vi "Status Steuerung.vi"() -> ()   [LabVIEW 2020, in "Erweiterte Konfig.lvlib"]
uses:
  Erweiterte Konfig.lvlib
  Visualisierungs Elemente/Button.ctl
  cRIO/Verwaltung/Digital Eingaenge 0-15.ctl
  cRIO/Verwaltung/Digital Ausgaenge 0-31.ctl
  cRIO/Verwaltung/Analog Eingaenge.ctl
  cRIO/Allgemein/CPU Status.ctl
  cRIO/Allgemein/CPU Speicher Auslastung.ctl
  cRIO/Verwaltung/Digital Ausgaenge 32-63.ctl
  cRIO/Verwaltung/TC Eingaenge.ctl
  <vilib>/Utility/miscctls.llb/LVRowAndColumnTypeDef.ctl
  System Load/VI SysLoad.vi
  cRIO/PC/Kommunikation mit cRIO.lvlib
  Allgemein/allgemeine Sub-VIs.lvlib
  System Load/System Load.lvlib
  cRIO/Verwaltung/Verwaltung - cRIO.lvlib
  cRIO/Allgemein/Allgemein.lvlib
panel:
  in  "Hauptregisterkarte":T1(tab)
  out "Digital In 2":string[][](table) caption="Digital In"
  out "Digital In":string[][](table)
  out "Digital Out 2":string[][](table) caption="Digital Out 1"
  out "Digital Out 1":string[][](table)
  out "Analog In 2":string[][](table) caption="Analog In"
  out "Analog In":string[][](table)
  out "TC In 2":string[][](table)
  out "TC In 1":string[][](table)
  out "PID":string[][](table)=[["Heizung Filter:"], ["Heizung Pumpe:"], ["Heizung HL zu Filter:"], ["Heizung HL zu FT-IR:"], ["HL zu FID:"], ["Reserve"], ["Heizleitung SP1:"], ["Heizleitung SP2:"], ["Flussregelung"], ["Reserve:"], [""], [""]]
  in  "Systemauslastung":T2
  in  "Registerkarte":T3(tab)
  out "DI":T4
  out "DO":T5
  out "DO 32-63":T6
  out "Analog Input":T7
  out "TC Eingänge":T8
  out "CPU Auslastung":T9 caption="CPU usage"
  out "CPU Speicher":T10 caption="CPU memory"
  out "PID Stellwerte":i16[](array[numeric]) caption="Controller Output"
  in  "ABBRECHEN":T2
  # "Status PLC"
  # "Heating filter:"
  # "Heating Pump:"
  # "Heating HL to filter:"
  # "Heating HL to FT-IR:"
  # "HL zu FID:"
  # "Reserve"
  # "Heizleitung SP1:"
  # "Heizleitung SP2:"
  # "Flussregelung"
  # "Option:"
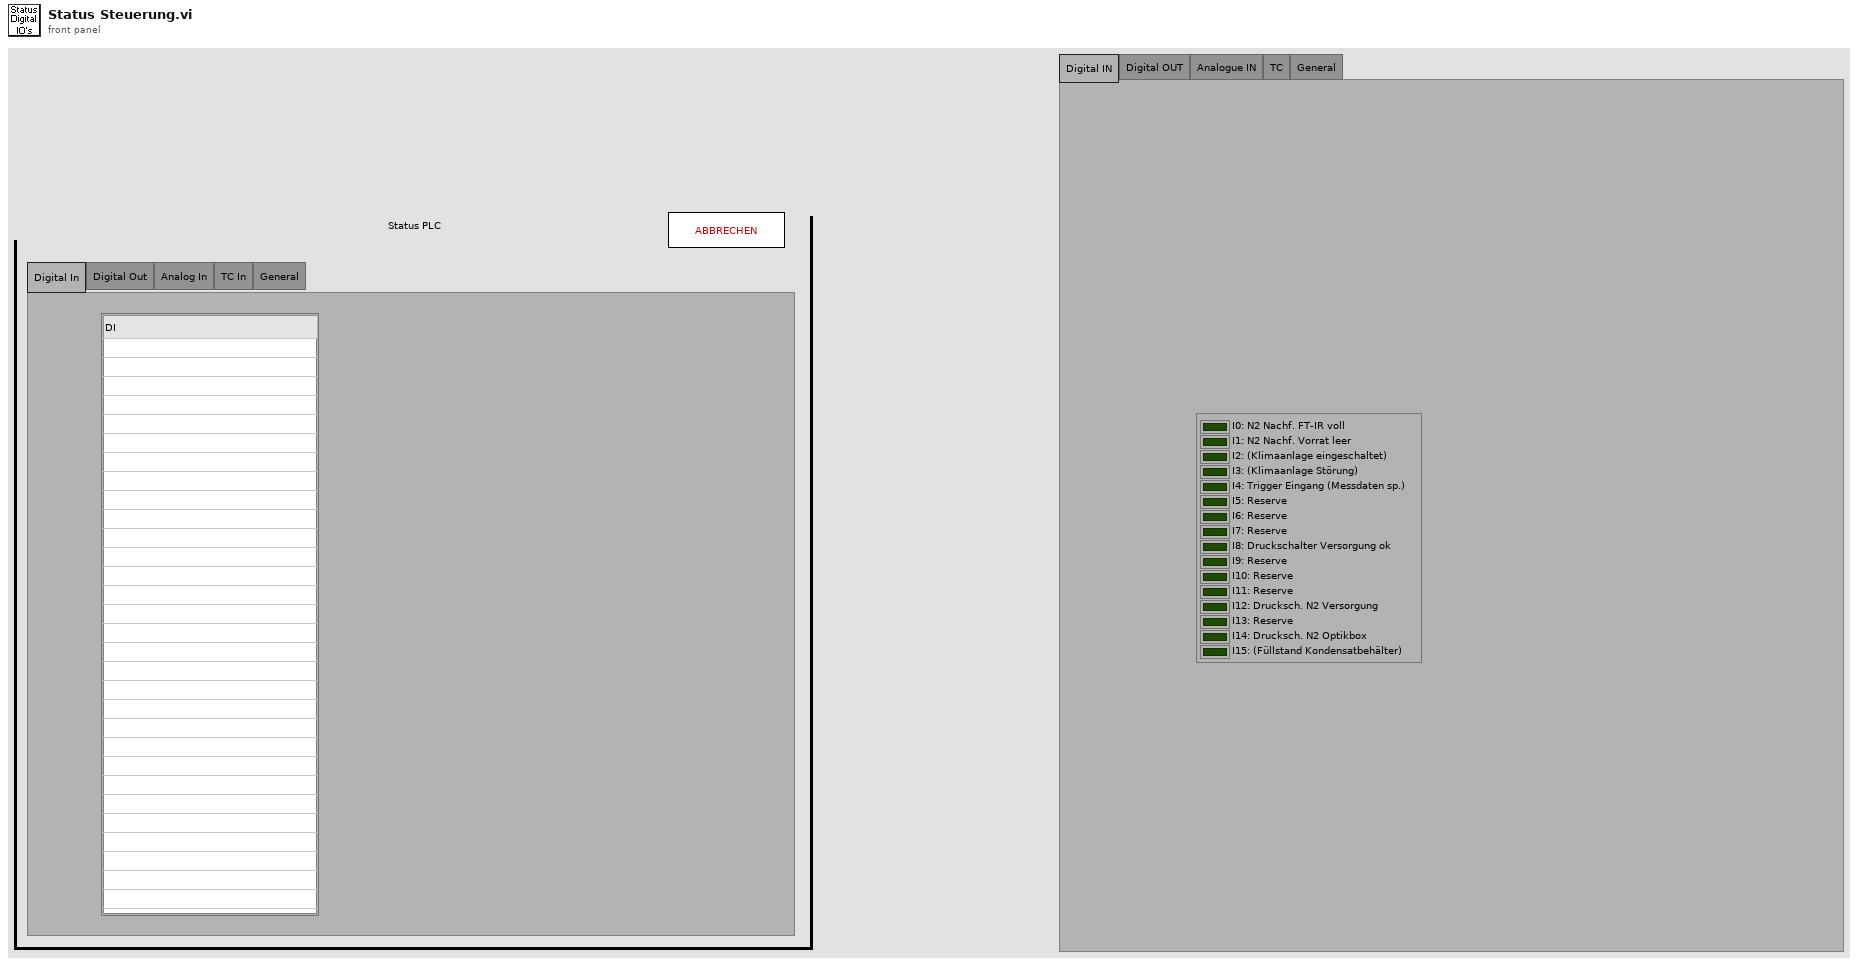
[diagram p1: front panel]
types:
  T1 = enum32{"Digital In", "Digital Out", "Analog In", "TC In", "General", "HovaCal Einstellungen"}
  T2 = typedef "Button.ctl" = bool
  T3 = enum32{"Digital IN", "Digital OUT", "Analogue IN", "TC", "General"}
  T4 = typedef "Verwaltung - cRIO.lvlib/Digital Eingaenge 0-15.ctl" = cluster{"I0: N2 Nachf. FT-IR voll":bool, "I1: N2 Nachf. Vorrat leer":bool, "I2: (Klimaanlage eingeschaltet)":bool, "I3: (Klimaanlage Störung)":bool, "I4: Trigger Eingang (Messdaten sp.)":bool, "I5: Reserve":bool, "I6: Reserve":bool, "I7: Reserve":bool, "I8: Druckschalter Versorgung ok":bool, "I9: Reserve":bool, "I10: Reserve":bool, "I11: Reserve":bool, "I12: Drucksch. N2 Versorgung":bool, "I13: Reserve":bool, "I14: Drucksch. N2 Optikbox":bool, "I15: (Füllstand Kondensatbehälter)":bool}
  T5 = typedef "Verwaltung - cRIO.lvlib/Digital Ausgaenge 0-31.ctl" = cluster{"O0: Druckluft Versorgung":bool, "O1: CG 1 (FB Eingang 1)":bool, "O2: CG 2 (Kühlung FT-IR EIN)":bool, "O3: CG 3 (FB Bypass)":bool, "O4: CG 4 (FB CalGas)":bool, "O5: CG 5 (FB spülen/UL)":bool, "O6: CG 6 (FB zum FT-IR)":bool, "O7: CG 7 (FB zum FID)":bool, "O8: CG 8 (FB Reserve)":bool, "O9: (FB Reserve)":bool, "O10: (FB Umgebungsluft FID)":bool, "O11: (FB zum Gaskühler)":bool, "O12: FB Stickstoff zu FT-IR":bool, "O13: Optikbox FT-IR spülen":bool, "O14: (Purifier deaktivieren)":bool, "O15: (Umschaltung Purifier/Stickstoff)":bool, "O16: N2 Einblasung":bool, "O17: LSP LN2 Nachfüllung":bool, "O18: (Reserve)":bool, "O19: (Pumpe Eingang1)":bool, "O20: (Pumpe Eingang2)":bool, "O21: (Pumpe Spülen1)":bool, "O22: (Pumpe Spülen2)":bool, "O23: (Reserve)":bool, "O24: CalGas 1":bool, "O25: CalGas 2":bool, "O26: CG 3-8 (CalGas 3)":bool, "O27: Stickstoff aufschalten":bool, "O28: CG zu PNS":bool, "O29: FTIR Standby Spülung":bool, "O30: CG zu Entnahme(T90)":bool, "O31: (Purifier regenerieren)":bool}
  T6 = typedef "Verwaltung - cRIO.lvlib/Digital Ausgaenge 32-63.ctl" = cluster{"O32: Messgaspumpe EIN":bool, "O33: (Umgebungsluftpumpe)":bool, "O34: (Kondensatpumpe GK)":bool, "O35: Klima/Lüfter EIN":bool, "O36: Versorgung Heizungen":bool, "O37: Versorgung Heizungen":bool, "O38: (Gaskühler EIN (Freigabe))":bool, "O39: Störung FAS LP":bool, "O40: (Heizung Filterblock)":bool, "O41: Heizung HL zu FT-IR":bool, "O42: Heizung HL Extern SP1":bool, "O43: Heizung HL Extern SP2":bool, "O44: Heizung Reserve":bool, "O45: Heizung Reserve":bool, "O46: Statusbeleuchtung grün":bool, "O47: Statusbeleuchtung rot":bool}
  T7 = typedef "Verwaltung - cRIO.lvlib/Analog Eingaenge.ctl" = cluster{"AI0: Durchfluss FT-IR":sgl, "AI1: Druck Ausgang":sgl, "AI2: Umgebungsdruck":sgl, "AI3: Druck FT-IR":sgl, "AI4: Druck CalGas":sgl, "AI5: Reserve":sgl, "AI6: Reserve":sgl, "AI7: Reserve":sgl, "Rohwert Durchfluss FT-IR":sgl, "Rohwert Druck Ausgang":sgl, "Rohwert Umgebungsdruck":sgl, "Rohwert Druck FT-IR":sgl, "Rohwert Druck CalGas":sgl, "Rohwert AI5":sgl, "Rohwert AI6":sgl, "Rohwert AI7":sgl, "Rohwert Diffdruck mbar FTIR":sgl}
  T8 = typedef "Verwaltung - cRIO.lvlib/TC Eingaenge.ctl" = cluster{"TC0: Reserve":sgl, "TC1: HL zu FT-IR":sgl, "TC2: HL Extern SP1":sgl, "TC3: HL Extern SP2":sgl, "TC4: Reserve":sgl, "TC5: Reserve":sgl, "TC6: Reserve":sgl, "TC7: Reserve":sgl, "TC8: FT-IR":sgl, "TC9: Reserve":sgl, "TC10: Schaltschrank":sgl, "TC11: Umgebung":sgl}
  T9 = typedef "Allgemein.lvlib/CPU Status.ctl" = cluster{"Total (%)":sgl, "Time Critical (%)":sgl, "Timed Structures (%)":sgl, "High (%)":sgl, "Above Normal (%)":sgl, "Normal (%)":sgl, "Background (%)":sgl, "Idle (%)":sgl, "ISR (%)":sgl}
  T10 = typedef "Allgemein.lvlib/CPU Speicher Auslastung.ctl" = cluster{"total (bytes)":u32, "available (bytes)":u32, "largest contiguous (bytes)":u32}
  T11 = typedef "LVRowAndColumnTypeDef.ctl" = cluster{"Row":i32, "Column":i32}
  T12 = cluster{"Numeric":sgl, "Numeric":sgl, "Numeric":sgl, "Numeric":sgl, "Numeric":sgl, "Numeric":sgl, "Numeric":sgl, "Numeric":sgl, "Numeric":sgl}
  T13 = cluster{"Numeric":sgl, "Numeric":sgl, "Numeric":sgl}
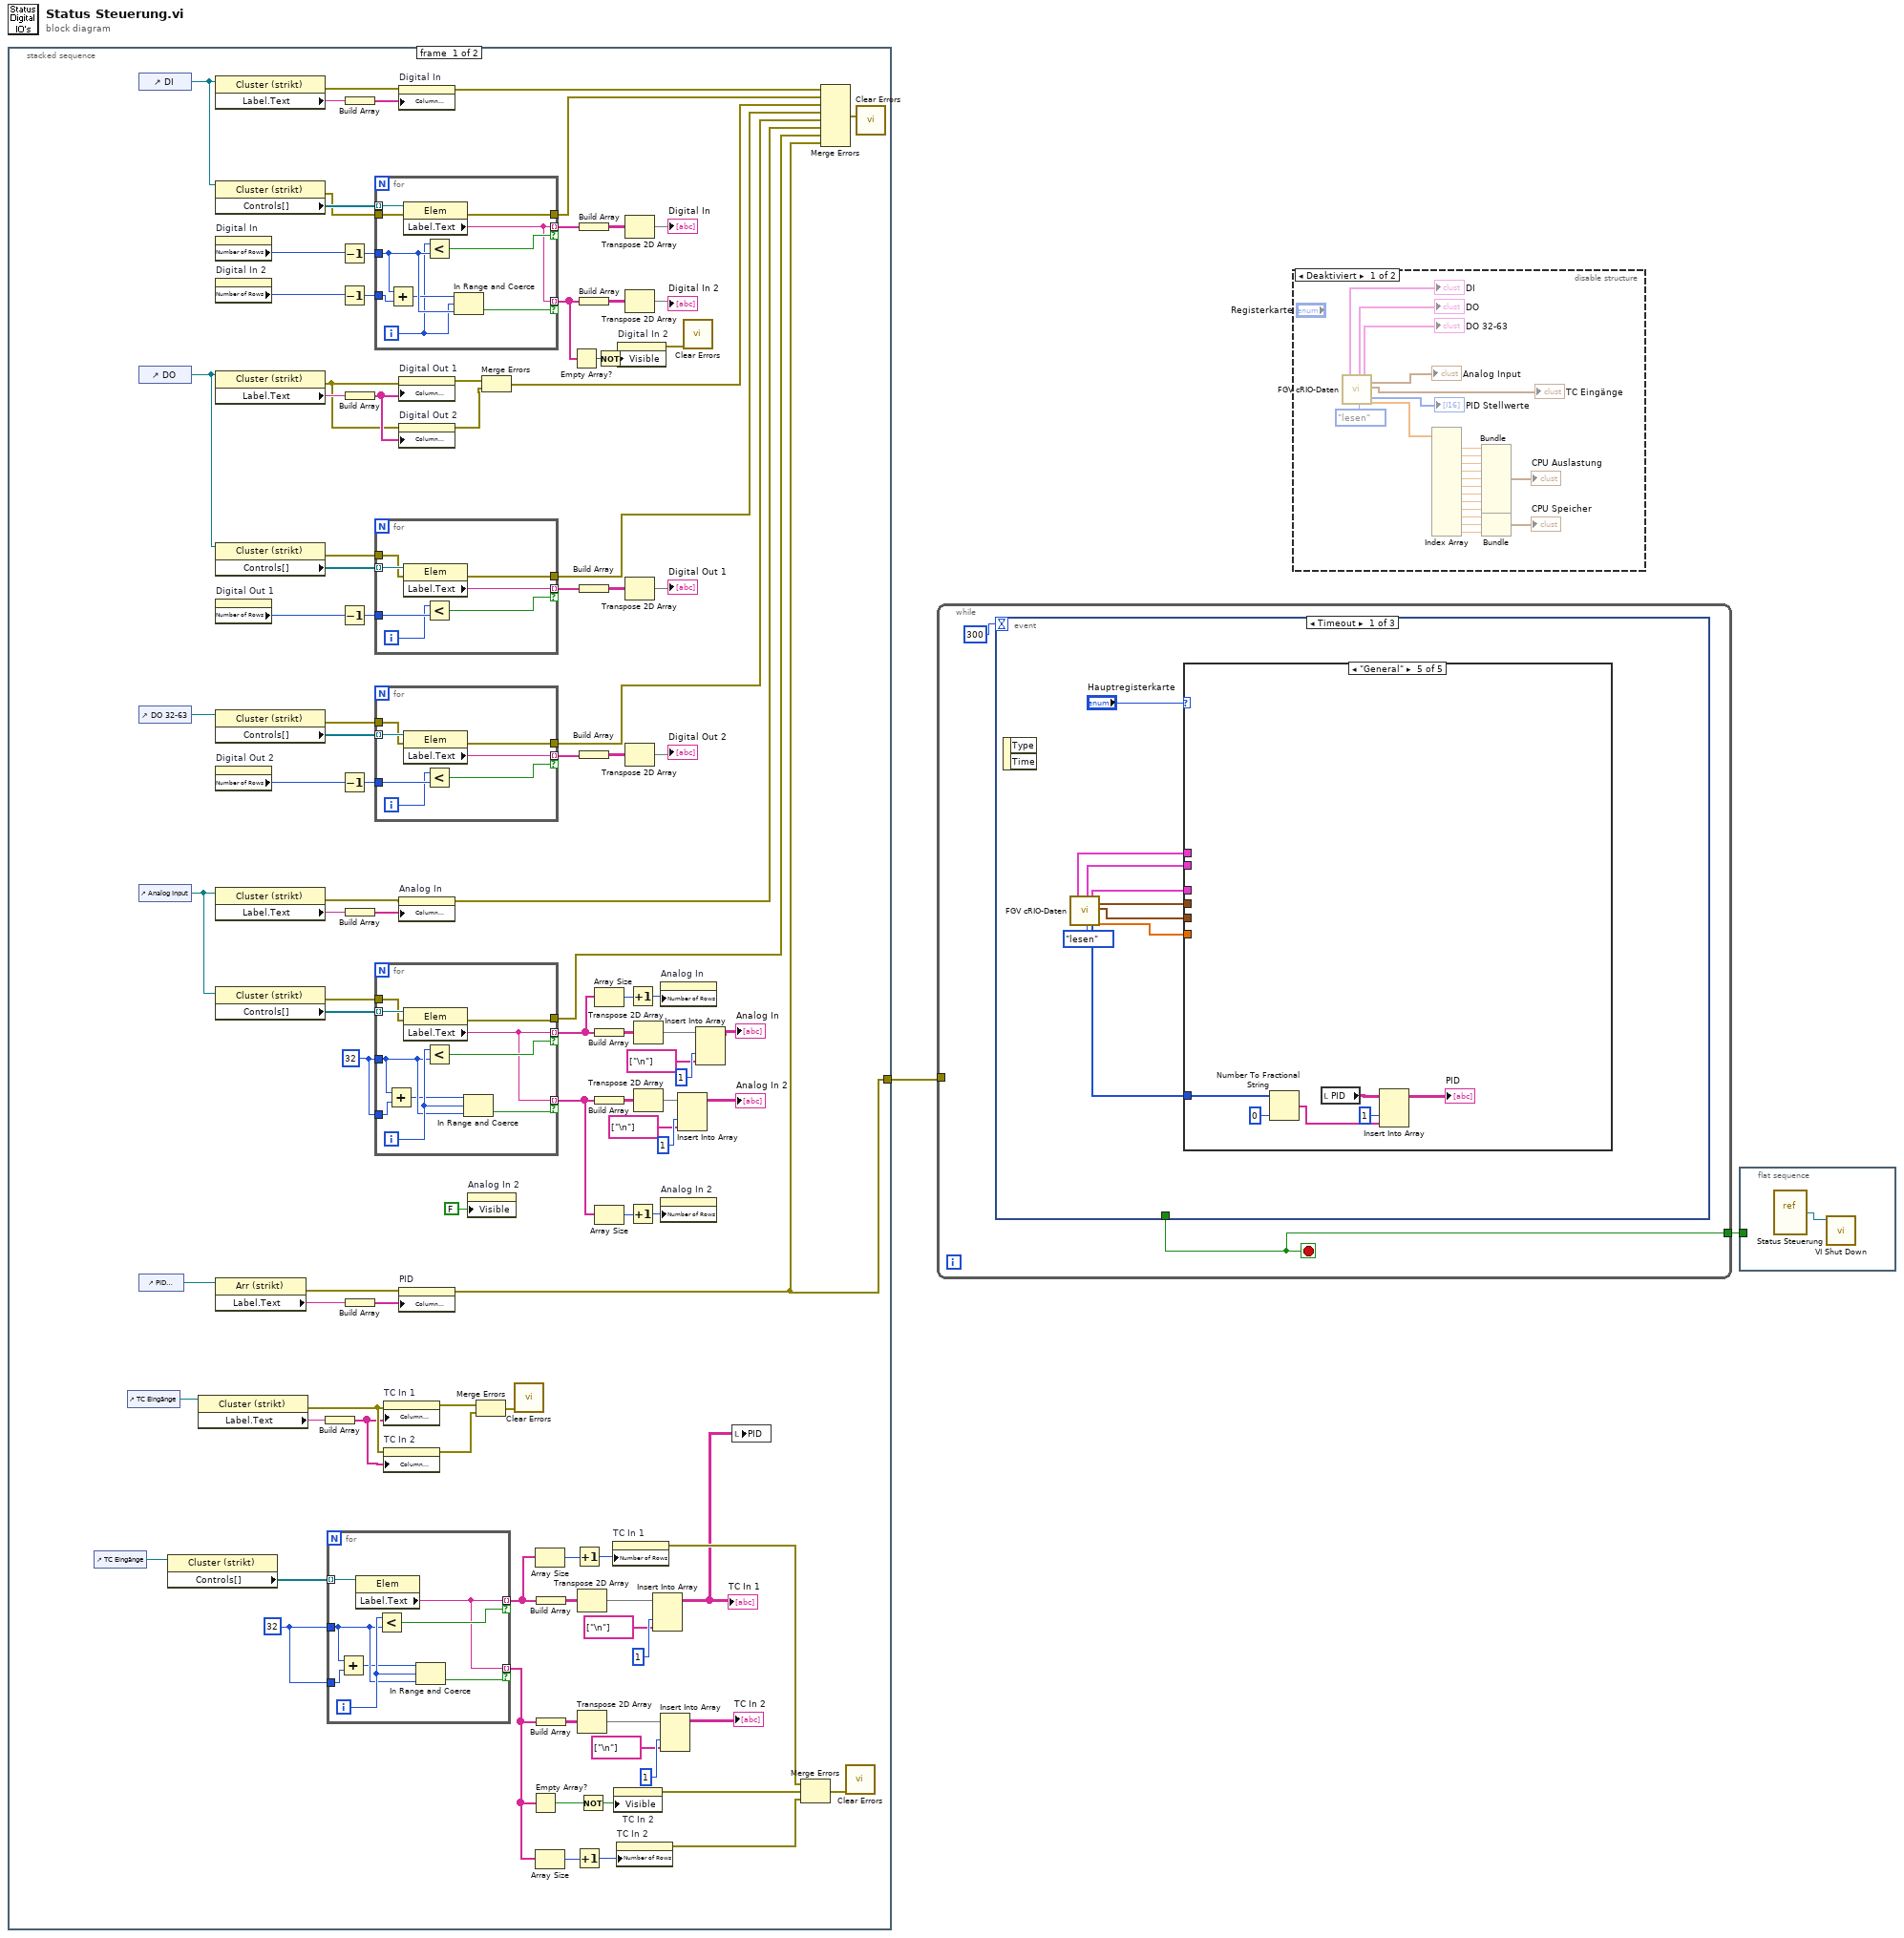
[diagram p0: block diagram]
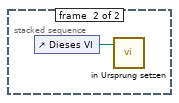
[diagram p3: hidden frame]
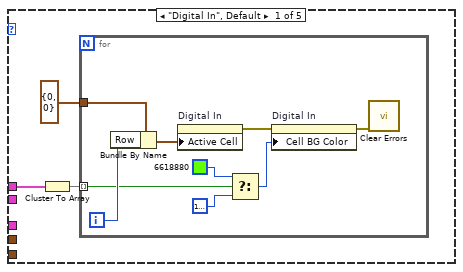
[diagram p4: hidden frame]
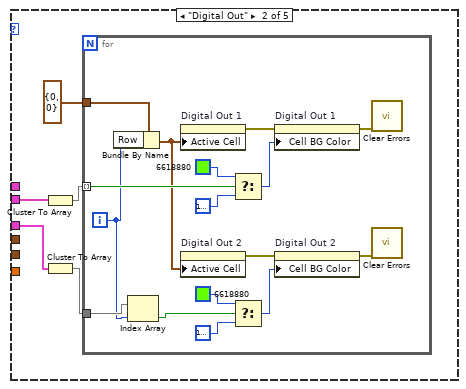
[diagram p5: hidden frame]
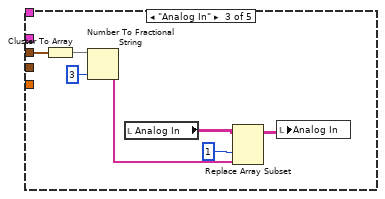
[diagram p6: hidden frame]
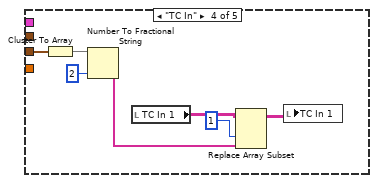
[diagram p7: hidden frame]
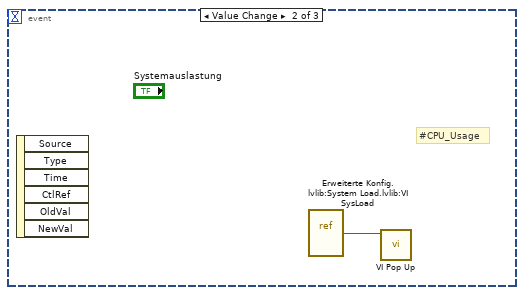
[diagram p8: hidden frame]
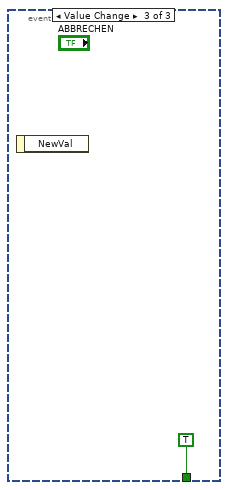
[diagram p9: hidden frame]
diagram:
  n1 = stacked-sequence {
    tunnel: [w5 _] -> w1
    frame #0 {
      w32 = u32 32 ("Zeilenanzahl")
      w43 = u32 32
      n2 = control-ref of="TC Eingänge"() -> (w74:refnum<vi>)
      n3 = control-ref of="TC Eingänge"() -> (w79:refnum<vi>)
      n4 = control-ref of="DI"() -> (w65:refnum<vi>)
      n5 = control-ref of="DO"() -> (w64:refnum<vi>)
      n6 = control-ref of="DO 32-63"() -> (w96:refnum<vi>)
      n7 = control-ref of="Analog Input"() -> (w63:refnum<vi>)
      n8 = control-ref of="PID Stellwerte"() -> (w66:refnum<vi>)
      n9 = property class="Cluster (strikt)"(reference=w74) -> ("Controls[]"=w76:refnum<vi>[])  [unwired: 1 in, 2 out]
      n10 = property class="Cluster (strikt)"(reference=w79) -> (error out=w81:errorcluster, "Label.Text"=w78:string)  [unwired: 1 in, 1 out]
      n11 = property class="Cluster (strikt)"(reference=w65) -> (error out=w89:errorcluster, "Label.Text"=w108:string)  [unwired: 1 in, 1 out]
      n12 = property class="Cluster (strikt)"(reference=w65) -> (error out=w62:errorcluster, "Controls[]"=w111:refnum<vi>[])  [unwired: 1 in, 1 out]
      n13 = property on="Digital In" class="Tbl (strikt)"() -> ("Number of Rows"=w90:u32)  [unwired: 2 in, 2 out]
      n14 = property on="Digital In 2" class="Tbl (strikt)"() -> ("Number of Rows"=w71:u32)  [unwired: 2 in, 2 out]
      n15 = property class="Cluster (strikt)"(reference=w64) -> (error out=w98:errorcluster, "Label.Text"=w106:string)  [unwired: 1 in, 1 out]
      n16 = property class="Cluster (strikt)"(reference=w64) -> (error out=w61:errorcluster, "Controls[]"=w101:refnum<vi>[])  [unwired: 1 in, 1 out]
      n17 = property on="Digital Out 1" class="Tbl (strikt)"() -> ("Number of Rows"=w104:u32)  [unwired: 2 in, 2 out]
      n18 = property class="Cluster (strikt)"(reference=w96) -> (error out=w60:errorcluster, "Controls[]"=w95:refnum<vi>[])  [unwired: 1 in, 1 out]
      n19 = property on="Digital Out 2" class="Tbl (strikt)"() -> ("Number of Rows"=w94:u32)  [unwired: 2 in, 2 out]
      n20 = property class="Cluster (strikt)"(reference=w63) -> (error out=w86:errorcluster, "Label.Text"=w85:string)  [unwired: 1 in, 1 out]
      n21 = property class="Cluster (strikt)"(reference=w63) -> (error out=w59:errorcluster, "Controls[]"=w83:refnum<vi>[])  [unwired: 1 in, 1 out]
      n22 = property class="Arr (strikt)"(reference=w66) -> (error out=w68:errorcluster, "Label.Text"=w69:string)  [unwired: 1 in, 1 out]
      n23 = Build Array(w78) -> (w80:string[])
      n24 = for {
        tunnel: w76 -> [w119] mode=indexing
        tunnel: [w113] -> w42 mode=indexing if=w118
        tunnel: w43 -> [w115]
        tunnel: w43 -> [w116]
        tunnel: [w113] -> w33 mode=indexing if=w112
        i -> [w117]
        n25 = Add(x=w115, y=w116) -> (x+y=w114:u32)
        n26 = property class="Elem"(reference=w119) -> ("Label.Text"=w113:string)  [unwired: 1 in, 2 out]
        n27 = Less?(x=w117, y=w115) -> (x < y?=w118:bool)
        n28 = In Range and Coerce(upper limit=w114, x=w117, lower limit=w115) -> (In Range?=w112:bool)  [unwired: 1 out]
      }
      n29 = Decrement(x=w90) -> (x-1=w107:u32)
      n30 = Decrement(x=w71) -> (x-1=w70:u32)
      n31 = Decrement(x=w104) -> (x-1=w105:u32)
      n32 = Decrement(x=w94) -> (x-1=w93:u32)
      n33 = Build Array(w108) -> (w88:string[])
      n34 = Build Array(w106) -> (w99:string[])
      n35 = Build Array(w85) -> (w87:string[])
      n36 = Build Array(w69) -> (w67:string[])
      n37 = for {
        tunnel: w111 -> [w153] mode=indexing
        tunnel: [w151] -> w110 mode=indexing if=w152
        tunnel: w107 -> [w148]
        tunnel: [w151] -> w49 mode=indexing if=w150
        tunnel: w70 -> [w149]
        tunnel: w62 -> [w145]
        tunnel: [w144] -> w57
        i -> [w146]
        n38 = Add(x=w148, y=w149) -> (x+y=w147:u32)
        n39 = property class="Elem"(reference=w153, error in=w145) -> (error out=w144:errorcluster, "Label.Text"=w151:string)  [unwired: 1 out]
        n40 = Less?(x=w146, y=w148) -> (x < y?=w152:bool)
        n41 = In Range and Coerce(upper limit=w147, x=w146, lower limit=w148) -> (In Range?=w150:bool)  [unwired: 1 out]
      }
      n42 = for {
        tunnel: w101 -> [w143] mode=indexing
        tunnel: [w142] -> w102 mode=indexing if=w141
        tunnel: w105 -> [w140]
        tunnel: w61 -> [w138]
        tunnel: [w137] -> w53
        i -> [w139]
        n43 = property class="Elem"(reference=w143, error in=w138) -> (error out=w137:errorcluster, "Label.Text"=w142:string)  [unwired: 1 out]
        n44 = Less?(x=w139, y=w140) -> (x < y?=w141:bool)
      }
      n45 = for {
        tunnel: w95 -> [w136] mode=indexing
        tunnel: [w135] -> w92 mode=indexing if=w134
        tunnel: w93 -> [w133]
        tunnel: w60 -> [w131]
        tunnel: [w130] -> w52
        i -> [w132]
        n46 = property class="Elem"(reference=w136, error in=w131) -> (error out=w130:errorcluster, "Label.Text"=w135:string)  [unwired: 1 out]
        n47 = Less?(x=w132, y=w133) -> (x < y?=w134:bool)
      }
      n48 = for {
        tunnel: w83 -> [w129] mode=indexing
        tunnel: [w123] -> w30 mode=indexing if=w128
        tunnel: w32 -> [w125]
        tunnel: w32 -> [w126]
        tunnel: [w123] -> w28 mode=indexing if=w122
        tunnel: w59 -> [w121]
        tunnel: [w120] -> w50
        i -> [w127]
        n49 = Add(x=w125, y=w126) -> (x+y=w124:u32)
        n50 = property class="Elem"(reference=w129, error in=w121) -> (error out=w120:errorcluster, "Label.Text"=w123:string)  [unwired: 1 out]
        n51 = Less?(x=w127, y=w125) -> (x < y?=w128:bool)
        n52 = In Range and Coerce(upper limit=w124, x=w127, lower limit=w125) -> (In Range?=w122:bool)  [unwired: 1 out]
      }
      n53 = property on="TC In 1" class="Tbl (strikt)"(error in=w81, "Column Headers[]"=w80) -> (error out=w24:errorcluster)  [unwired: 1 in, 1 out]
      n54 = property on="TC In 2" class="Tbl (strikt)"(error in=w81, "Column Headers[]"=w80) -> (error out=w23:errorcluster)  [unwired: 1 in, 1 out]
      n55 = property on="Digital In" class="Tbl (strikt)"(error in=w89, "Column Headers[]"=w88) -> (error out=w58:errorcluster)  [unwired: 1 in, 1 out]
      n56 = property on="Digital Out 1" class="Tbl (strikt)"(error in=w98, "Column Headers[]"=w99) -> (error out=w56:errorcluster)  [unwired: 1 in, 1 out]
      n57 = property on="Digital Out 2" class="Tbl (strikt)"(error in=w98, "Column Headers[]"=w99) -> (error out=w55:errorcluster)  [unwired: 1 in, 1 out]
      n58 = property on="Analog In" class="Tbl (strikt)"(error in=w86, "Column Headers[]"=w87) -> (error out=w51:errorcluster)  [unwired: 1 in, 1 out]
      n59 = property on="PID" class="Tbl (strikt)"(error in=w68, "Column Headers[]"=w67) -> (error out=w5:errorcluster)  [unwired: 1 in, 1 out]
      n60 = property on="Analog In 2" class="Tbl (strikt)"("Visible"=FALSE ("Sichtbar")) -> ()  [unwired: 2 in, 2 out]
      n61 = Merge Errors(w24, w23) -> (w22:errorcluster)
      n62 = Merge Errors(w56, w55) -> (w54:errorcluster)
      n63 = call <vilib>:"Clear Errors.vi"("error in (no error)"=w22) -> ()  [unwired: 5 in, 2 out]
      n64 = Empty Array?(array=w33) -> (empty?=w45:bool)
      n65 = Array Size(array=w42) -> (size(s)=w41:i32)
      n66 = Array Size(array=w33) -> (size(s)=w35:i32)
      n67 = Build Array(w42) -> (w75:string[][])
      n68 = Build Array(w33) -> (w77:string[][])
      n69 = Empty Array?(array=w49) -> (empty?=w48:bool)
      n70 = Increment(x=w41) -> (x+1=w40:i32)
      n71 = Increment(x=w35) -> (x+1=w34:i32)
      n72 = Transpose 2D Array(2D array=w75) -> (transposed array=w10:string[][])
      n73 = Transpose 2D Array(2D array=w77) -> (transposed array=w7:string[][])
      n74 = Not(x=w45) -> (.not. x?=w44:bool)
      n75 = Build Array(w110) -> (w109:string[][])
      n76 = Build Array(w49) -> (w73:string[][])
      n77 = Build Array(w102) -> (w103:string[][])
      n78 = Build Array(w92) -> (w97:string[][])
      n79 = Array Size(array=w30) -> (size(s)=w31:i32)
      n80 = Build Array(w30) -> (w84:string[][])
      n81 = Build Array(w28) -> (w82:string[][])
      n82 = Array Size(array=w28) -> (size(s)=w29:i32)
      n83 = Not(x=w48) -> (.not. x?=w46:bool)
      n84 = property on="TC In 1" class="Tbl (strikt)"("Number of Rows"=w40) -> (error out=w38:errorcluster)  [unwired: 2 in, 1 out]
      n85 = property on="TC In 2" class="Tbl (strikt)"("Visible"=w44) -> (error out=w37:errorcluster)  [unwired: 2 in, 1 out]
      n86 = property on="TC In 2" class="Tbl (strikt)"("Number of Rows"=w34) -> (error out=w36:errorcluster)  [unwired: 2 in, 1 out]
      n87 = property on="Digital In 2" class="Tbl (strikt)"("Visible"=w46) -> (error out=w47:errorcluster)  [unwired: 2 in, 1 out]
      n88 = Transpose 2D Array(2D array=w109) -> (transposed array=→"Digital In":string[][])
      n89 = Transpose 2D Array(2D array=w73) -> (transposed array=→"Digital In 2":string[][])
      n90 = Transpose 2D Array(2D array=w103) -> (transposed array=→"Digital Out 1":string[][])
      n91 = Transpose 2D Array(2D array=w97) -> (transposed array=→"Digital Out 2":string[][])
      n92 = Increment(x=w31) -> (x+1=w26:i32)
      n93 = Increment(x=w29) -> (x+1=w27:i32)
      n94 = Transpose 2D Array(2D array=w84) -> (transposed array=w17:string[][])
      n95 = Transpose 2D Array(2D array=w82) -> (transposed array=w14:string[][])
      n96 = Insert Into Array(array=w10, index (col)=1 ("Deaktivierter Index (Spalte)"), new element=string[] ["\n"] ("Neues Element/Teil-Array")) -> (w3:string[][])  [unwired: 1 in]
      "TC In 1" <- w3
      n97 = property on="Analog In" class="Tbl (strikt)"("Number of Rows"=w26) -> ()  [unwired: 2 in, 2 out]
      n98 = property on="Analog In 2" class="Tbl (strikt)"("Number of Rows"=w27) -> ()  [unwired: 2 in, 2 out]
      n99 = Insert Into Array(array=w7, index (col)=1 ("Deaktivierter Index (Spalte)"), new element=string[] ["\n"] ("Neues Element/Teil-Array")) -> (→"TC In 2":string[][])  [unwired: 1 in]
      n100 = Insert Into Array(array=w14, index (col)=1 ("Deaktivierter Index (Spalte)"), new element=string[] ["\n"] ("Neues Element/Teil-Array")) -> (→"Analog In 2":string[][])  [unwired: 1 in]
      n101 = call <vilib>:"Clear Errors.vi"("error in (no error)"=w47) -> ()  [unwired: 5 in, 2 out]
      n102 = Insert Into Array(array=w17, index (col)=1 ("Deaktivierter Index (Spalte)"), new element=string[] ["\n"] ("Neues Element/Teil-Array")) -> (→"Analog In":string[][])  [unwired: 1 in]
      n103 = local write "PID"(w3) -> ()
      n104 = Merge Errors(w38, w37, w36) -> (w39:errorcluster)
      n105 = Merge Errors(w58, w57, w54, w53, w52, w51, w50, w5) -> (w21:errorcluster)
      n106 = call <vilib>:"Clear Errors.vi"("error in (no error)"=w39) -> ()  [unwired: 5 in, 2 out]
      n107 = call <vilib>:"Clear Errors.vi"("error in (no error)"=w21) -> ()  [unwired: 5 in, 2 out]
    }
    frame #1 {
      n108 = control-ref of="Dieses VI"() -> (w154:refnum<vi>)
      n109 = call "in Ursprung setzen.vi"("VI Referenz"=w154) -> ()  [unwired: 10 in, 1 out]
    }
  }
  n110 = while {
    tunnel: [w155] -> w2
    tunnel: w1 -> [_]
    stop <- w155 stop-if-true
    n111 = event shown="[0] Timeout" {
      selector: _ -> [_ _ _]
      dyn-events: _ -> [_ _ _]
      timeout: 300 -> [_ _ _]
      tunnel: [_ _ TRUE ("ABBRECHEN")] -> w155
      event Timeout {
        n112 = event-data() -> ()  [unwired: 1 in, 2 out]
        n113 = call "FGV cRIO-Daten.vi"("Aktion"=enum16{"lesen", "schreiben"}."lesen") -> ("DI"=w161:T4, "DO 0-31"=w162:T5, "DO 32-63"=w163:T6, "PID Stellwerte"=w157:i16[], "Analog Input"=w164:T7, "TC Eingänge"=w165:T8, "CPU Status"=w158:sgl[])  [unwired: 9 in, 3 out]
        n114 = case shown="\"General\"" "Hauptregisterkarte" {
          tunnel: w161 -> [w168 _ _ _ _]
          tunnel: w162 -> [_ w180 _ _ _]
          tunnel: w163 -> [_ w179 _ _ _]
          tunnel: w164 -> [_ _ w205 _ _]
          tunnel: w165 -> [_ _ _ w211 _]
          tunnel: w158 -> [_ _ _ _ _]
          tunnel: w157 -> [_ _ _ _ w218]
          frame "Digital In", Default {
            n115 = Cluster To Array(cluster=w168) -> (array=w167:bool[])
            n116 = for {
              tunnel: w167 -> [w173] mode=indexing
              tunnel: T11 {"Row"=0, "Column"=0} ("Aktive Zelle:Aktive Zelle") -> [w177]
              i -> [w176]
              n117 = Bundle By Name(cluster=w177, "Row"=w176) -> (w175:T11)
              n118 = property on="Digital In" class="Tbl (strikt)"("Active Cell"=w175) -> (error out=w174:errorcluster)  [unwired: 2 in, 1 out]
              n119 = Select(t=u32 6618880, s=w173, f=u32 16777225) -> (s? t:f=w172:u32)
              n120 = property on="Digital In" class="Tbl (strikt)"(error in=w174, "Cell BG Color"=w172) -> (error out=w171:errorcluster)  [unwired: 1 in, 1 out]
              n121 = call <vilib>:"Clear Errors.vi"("error in (no error)"=w171) -> ()  [unwired: 5 in, 2 out]
            }
          }
          frame "Digital Out" {
            n122 = Cluster To Array(cluster=w180) -> (array=w181:bool[])
            n123 = Cluster To Array(cluster=w179) -> (array=w178:bool[])
            n124 = for {
              tunnel: w181 -> [w192] mode=indexing
              tunnel: T11 {"Row"=0, "Column"=0} ("Aktive Zelle:Aktive Zelle") -> [w198]
              tunnel: w178 -> [w185]
              i -> [w183]
              n125 = Bundle By Name(cluster=w198, "Row"=w183) -> (w186:T11)
              n126 = Index Array(array=w185, index=w183) -> (element=w184:bool)
              n127 = property on="Digital Out 1" class="Tbl (strikt)"("Active Cell"=w186) -> (error out=w197:errorcluster)  [unwired: 2 in, 1 out]
              n128 = property on="Digital Out 2" class="Tbl (strikt)"("Active Cell"=w186) -> (error out=w187:errorcluster)  [unwired: 2 in, 1 out]
              n129 = Select(t=u32 6618880, s=w192, f=u32 16777225) -> (s? t:f=w196:u32)
              n130 = Select(t=u32 6618880, s=w184, f=u32 16777225) -> (s? t:f=w188:u32)
              n131 = property on="Digital Out 1" class="Tbl (strikt)"(error in=w197, "Cell BG Color"=w196) -> (error out=w195:errorcluster)  [unwired: 1 in, 1 out]
              n132 = property on="Digital Out 2" class="Tbl (strikt)"(error in=w187, "Cell BG Color"=w188) -> (error out=w189:errorcluster)  [unwired: 1 in, 1 out]
              n133 = call <vilib>:"Clear Errors.vi"("error in (no error)"=w195) -> ()  [unwired: 5 in, 2 out]
              n134 = call <vilib>:"Clear Errors.vi"("error in (no error)"=w189) -> ()  [unwired: 5 in, 2 out]
            }
          }
          frame "Analog In" {
            n135 = Cluster To Array(cluster=w205) -> (array=w204:sgl[])
            n136 = Number To Fractional String(number=w204, precision (6)=i16 3 ("Genauigkeit (6)")) -> (F-format string=w199:string[])  [unwired: 2 in]
            n137 = local read "Analog In"() -> (w200:string[][])
            n138 = Replace Array Subset(array=w200, new element=w199, index (col)=1 ("Deaktivierter Index (Spalte)")) -> (w201:string[][])  [unwired: 1 in]
            n139 = local write "Analog In"(w201) -> ()
          }
          frame "TC In" {
            n140 = Cluster To Array(cluster=w211) -> (array=w212:sgl[])
            n141 = Number To Fractional String(number=w212, precision (6)=i16 2 ("Genauigkeit (6)")) -> (F-format string=w206:string[])  [unwired: 2 in]
            n142 = local read "TC In 1"() -> (w208:string[][])
            n143 = Replace Array Subset(array=w208, new element=w206, index (col)=1 ("Deaktivierter Index (Spalte)")) -> (w207:string[][])  [unwired: 1 in]
            n144 = local write "TC In 1"(w207) -> ()
          }
          frame "General" {
            n145 = Number To Fractional String(number=w218, precision (6)=i16 0 ("Genauigkeit (6)")) -> (F-format string=w214:string[])  [unwired: 2 in]
            n146 = local read "PID"() -> (w216:string[][])
            n147 = Insert Into Array(array=w216, index (col)=1 ("Deaktivierter Index (Spalte)"), new element=w214) -> (→"PID":string[][])  [unwired: 1 in]
          }
        }
      }
      event Value Change {
        # "#CPU_Usage"
        n148 = event-data() -> ()  [unwired: 1 in, 6 out]
        n149 = vi-ref "Erweiterte Konfig.lvlib:System Load.lvlib:VI SysLoad.vi"() -> (w219:refnum<vi>)
        n150 = call "VI Pop Up.vi"("VI Referenz"=w219) -> ()  [unwired: 10 in, 1 out]
      }
      event Value Change {
        n151 = event-data() -> ()  [unwired: 1 in, 1 out]
      }
    }
  }
  n152 = disable-structure shown="Deaktiviert" {
    frame Disabled {
      n153 = call "FGV cRIO-Daten.vi"("Aktion"=enum16{"lesen", "schreiben"}."lesen") -> ("DI"=→"DI":T4, "DO 0-31"=→"DO":T5, "DO 32-63"=→"DO 32-63":T6, "PID Stellwerte"=→"PID Stellwerte":i16[], "Analog Input"=→"Analog Input":T7, "TC Eingänge"=→"TC Eingänge":T8, "CPU Status"=w240:sgl[])  [unwired: 9 in, 3 out]
      n154 = Index Array(array=w240) -> (element #1=w239:sgl, element #2=w238:sgl, element #3=w237:sgl, element #4=w236:sgl, element #5=w235:sgl, element #6=w234:sgl, element #7=w233:sgl, element #8=w232:sgl, element #9=w231:sgl, element #10=w229:sgl, element #11=w228:sgl, element #12=w227:sgl)  [unwired: 12 in]
      n155 = Bundle("Numeric"=w239, "Numeric"=w238, "Numeric"=w237, "Numeric"=w236, "Numeric"=w235, "Numeric"=w234, "Numeric"=w233, "Numeric"=w232, "Numeric"=w231) -> (→"CPU Auslastung":T12)  [unwired: 1 in]
      n156 = Bundle("Numeric"=w229, "Numeric"=w228, "Numeric"=w227) -> (→"CPU Speicher":T13)  [unwired: 1 in]
    }
    frame Enabled {
    }
  }
  n157 = flat-sequence {
    tunnel: w2 -> [_]
    frame #0 {
      n158 = vi-ref "Status Steuerung.vi"() -> (w243:refnum<vi>)
      n159 = call "VI Shut Down.vi"("VI Referenz"=w243) -> ()  [unwired: 11 in]
    }
  }
